vi "savedata.vi"() -> ()   [LabVIEW 2011]
uses:
  <vilib>/Utility/file.llb/Write To Spreadsheet File (DBL).vi
panel:
  out "Filtered data":dbl[](array[numeric])
  in  "Distance (cm)":dbl
  in  "num pts to avg":i32
  in  "Record button":bool
  out "Waveform Chart":T1(graph)
  in  "Log file":path
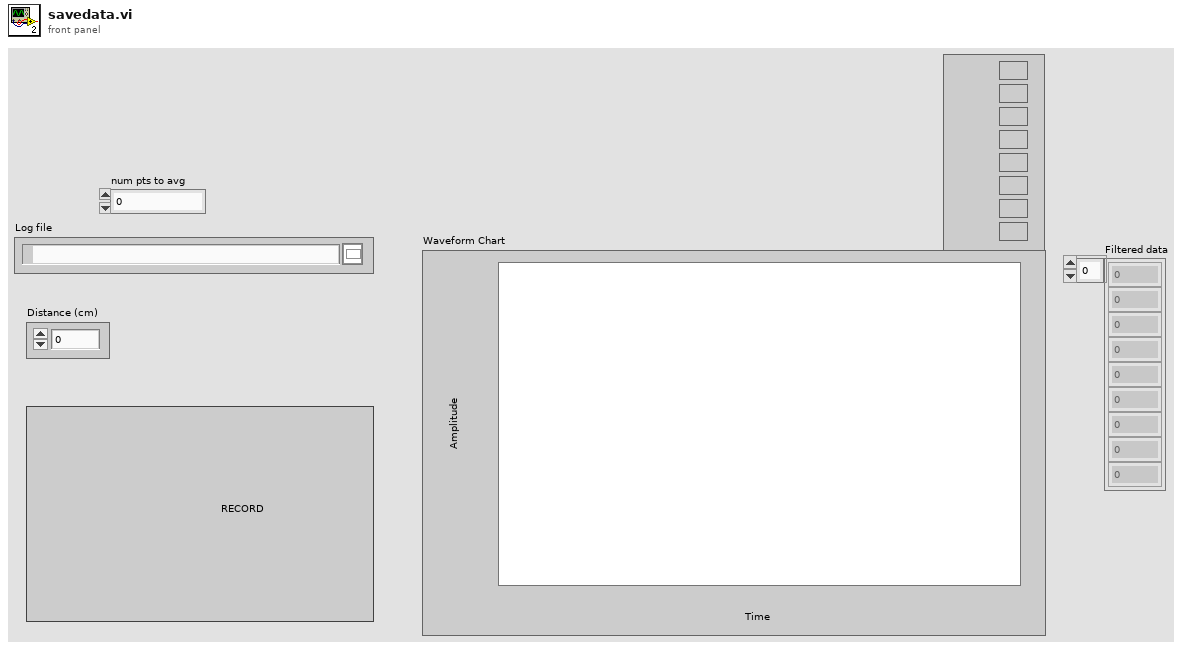
[diagram p1: front panel]
types:
  T1 = cluster{"[0]":dbl, "[1]":dbl, "[2]":dbl, "[3]":dbl, "[4]":dbl, "[5]":dbl, "[6]":dbl, "[7]":dbl, "[8]":dbl}
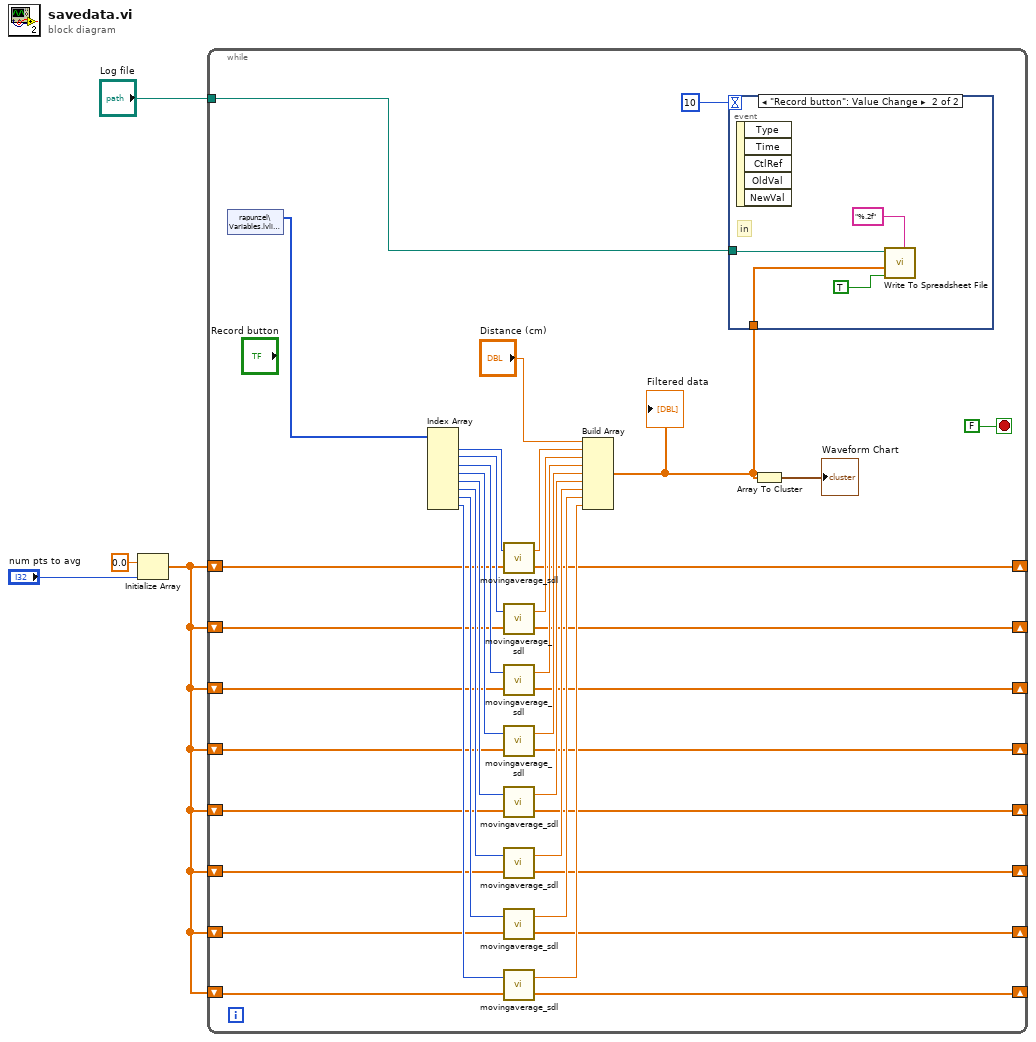
[diagram p0: block diagram]
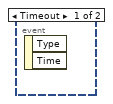
[diagram p2: hidden frame]
diagram:
  n1 = Initialize Array(0.0 ("element"), "num pts to avg") -> (w1:dbl[])
  n2 = while {
    tunnel: "Log file" -> [w42]
    shift-right: [w13] -> _
    shift-left: w1 -> [w21]
    shift-right: [w12] -> _
    shift-left: w1 -> [w20]
    shift-right: [w11] -> _
    shift-left: w1 -> [w19]
    shift-right: [w10] -> _
    shift-left: w1 -> [w18]
    shift-right: [w9] -> _
    shift-left: w1 -> [w17]
    shift-right: [w8] -> _
    shift-left: w1 -> [w16]
    shift-right: [w7] -> _
    shift-left: w1 -> [w15]
    shift-right: [w6] -> _
    shift-left: w1 -> [w14]
    stop <- FALSE stop-if-true
    n3 = shared-variable "rapunzel\\Variables.lvlib\\AI"() -> (w40:u16[])  [unwired: 1 in, 1 out]
    n4 = Index Array(array=w40) -> (element #1=w37:u16, element #2=w36:u16, element #3=w35:u16, element #4=w34:u16, element #5=w33:u16, element #6=w32:u16, element #7=w31:u16, element #8=w30:u16)  [unwired: 8 in]
    n5 = call "movingaverage_sdl.vi"("input array"=w21, "new element"=w37) -> ("Array"=w13:dbl[], "avg"=w29:dbl)
    n6 = call "movingaverage_sdl.vi"("input array"=w20, "new element"=w36) -> ("Array"=w12:dbl[], "avg"=w28:dbl)
    n7 = call "movingaverage_sdl.vi"("input array"=w19, "new element"=w35) -> ("Array"=w11:dbl[], "avg"=w27:dbl)
    n8 = call "movingaverage_sdl.vi"("input array"=w18, "new element"=w34) -> ("Array"=w10:dbl[], "avg"=w26:dbl)
    n9 = call "movingaverage_sdl.vi"("input array"=w17, "new element"=w33) -> ("Array"=w9:dbl[], "avg"=w25:dbl)
    n10 = call "movingaverage_sdl.vi"("input array"=w16, "new element"=w32) -> ("Array"=w8:dbl[], "avg"=w24:dbl)
    n11 = call "movingaverage_sdl.vi"("input array"=w15, "new element"=w31) -> ("Array"=w7:dbl[], "avg"=w23:dbl)
    n12 = call "movingaverage_sdl.vi"("input array"=w14, "new element"=w30) -> ("Array"=w6:dbl[], "avg"=w22:dbl)
    n13 = Build Array("Distance (cm)", w29, w28, w27, w26, w25, w24, w23, w22) -> (w38:dbl[])
    "Filtered data" <- w38
    n14 = event shown="[1] \"Record button\": Value Change" {
      selector: _ -> [_ _]
      dyn-events: _ -> [_ _]
      timeout: 10 -> [_ _]
      tunnel: w42 -> [_ w45]
      tunnel: w38 -> [_ w44]
      event Timeout {
        n15 = event-data() -> ()  [unwired: 1 in, 2 out]
      }
      event "Record button": Value Change {
        # "in"
        n16 = event-data() -> ()  [unwired: 1 in, 5 out]
        n17 = call-poly <vilib>:"Write To Spreadsheet File.vi"("format (%.3f)"="%.2f", "append to file? (new file:F)"=TRUE, "1D data"=w44, "file path (dialog if empty)"=w45) -> ()  [unwired: 4 in, 1 out]
      }
    }
    n18 = Array To Cluster(array=w38) -> (cluster=→"Waveform Chart":T1)
  }
